vi "Bit_statistics.vi"(5 "Write Code":u8[](array[numeric]) format="%b", 7 "Read Code":u8[](array[numeric]) format="%b") -> (0 "TotalErrorAddress":i32, 1 "TotalErrorBitsAddr":i32[](array[numeric]), 2 "TotalErrorBits":i32, 3 "Address Error":i32[](array[numeric]))   [LabVIEW 2018]
panel:
  out "size(s)":i32
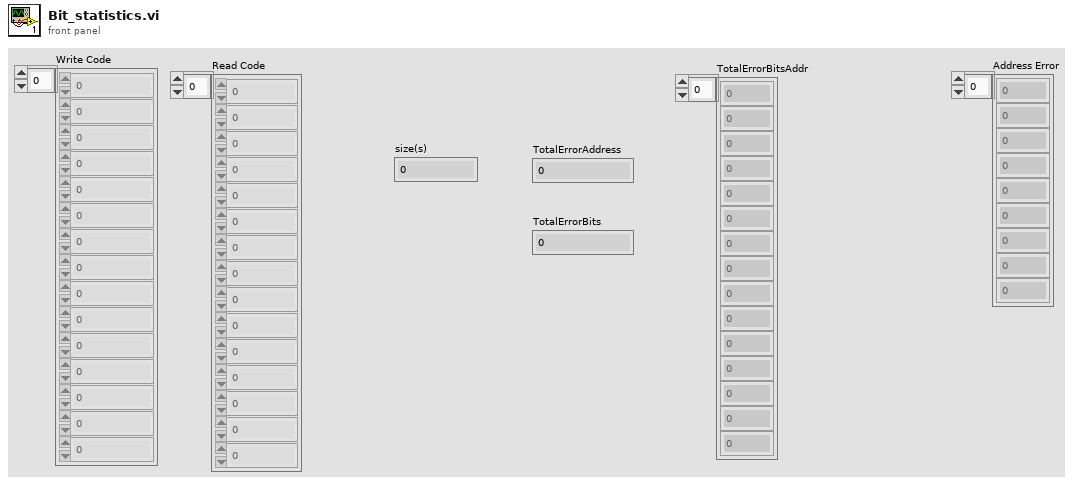
[diagram p1: front panel]
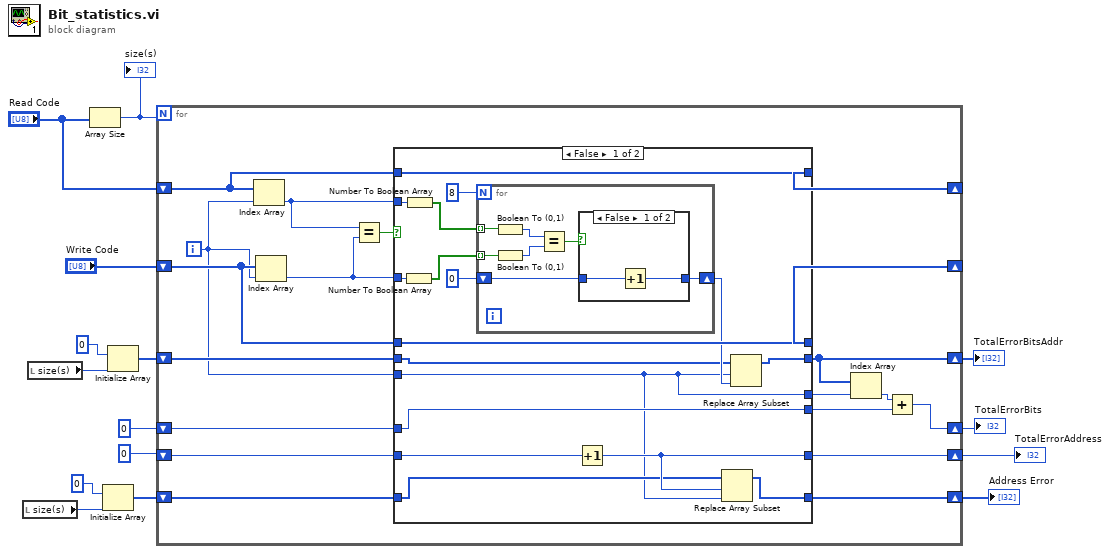
[diagram p0: block diagram]
diagram:
  n1 = local read "size(s)"() -> (w3:i32)
  n2 = local read "size(s)"() -> (w5:i32)
  n3 = Array Size(array="Read Code") -> (size(s)=w15:i32)
  "size(s)" <- w15
  n4 = Initialize Array(0 ("element"), w3) -> (w1:i32[])
  n5 = Initialize Array(0 ("element"), w5) -> (w11:i32[])
  n6 = for {
    N: w15 -> [_]
    shift-right: [w30] -> _
    shift-left: "Read Code" -> [w31]
    shift-right: [w28] -> _
    shift-left: "Write Code" -> [w29]
    shift-right: [w23] -> w8
    shift-left: w11 -> [w27]
    shift-right: [w25] -> w9
    shift-left: 0 ("element") -> [w26]
    shift-right: [w19] -> w6
    shift-left: 0 ("element") -> [w21]
    shift-right: [w16] -> w4
    shift-left: w1 -> [w17]
    i -> [w24]
    n7 = Index Array(array=w31, index=w24) -> (element=w33:u8)
    n8 = Index Array(array=w29, index=w24) -> (element=w32:u8)
    n9 = Equal?(x=w33, y=w32) -> (x = y?=w34:bool)
    n10 = case shown="False" w34 {
      tunnel: w33 -> [w49 _]
      tunnel: w32 -> [w48 _]
      tunnel: w31 -> [w51 w68]
      tunnel: [w51 w68] -> w30
      tunnel: w29 -> [w50 w67]
      tunnel: [w50 w67] -> w28
      tunnel: w27 -> [w42 w66]
      tunnel: [w41 w66] -> w23
      tunnel: w26 -> [w39 w64]
      tunnel: [w37 w64] -> w25
      tunnel: w24 -> [w35 w63]
      tunnel: [w35 w63] -> w22
      tunnel: w21 -> [w40 w65]
      tunnel: [w40 w65] -> w18
      tunnel: w17 -> [w36 w62]
      tunnel: [w38 w62] -> w16
      frame False {
        n11 = Number To Boolean Array(number=w48) -> (Boolean array=w45:bool[])
        n12 = Number To Boolean Array(number=w49) -> (Boolean array=w46:bool[])
        n13 = for {
          N: 8 -> [_]
          tunnel: w46 -> [w58] mode=indexing
          tunnel: w45 -> [w57] mode=indexing
          shift-right: [w52] -> w43
          shift-left: 0 -> [w53]
          n14 = Boolean To (0,1)(Boolean=w58) -> (0, 1=w56:i16)
          n15 = Boolean To (0,1)(Boolean=w57) -> (0, 1=w55:i16)
          n16 = Equal?(x=w56, y=w55) -> (x = y?=w54:bool)
          n17 = case shown="False" w54 {
            tunnel: w53 -> [w60 w61]
            tunnel: [w59 w61] -> w52
            frame False {
              n18 = Increment(x=w60) -> (x+1=w59:i32)
            }
            frame True {
            }
          }
        }
        n19 = Increment(x=w39) -> (x+1=w37:i32)
        n20 = Replace Array Subset(array=w36, new element=w35, index=w37) -> (w38:i32[])
        n21 = Replace Array Subset(array=w42, new element=w43, index=w35) -> (w41:i32[])
      }
      frame True {
      }
    }
    n22 = Index Array(array=w23, index=w22) -> (element=w20:i32)
    n23 = Add(x=w20, y=w18) -> (x+y=w19:i32)
  }
  "TotalErrorAddress" <- w9
  "TotalErrorBitsAddr" <- w8
  "TotalErrorBits" <- w6
  "Address Error" <- w4
